vi "Fit Color - Parabolic.vi"(9 "Height":i16, 10 "Color Shadow":u8, 11 "Color Hilite":u8) -> (3 "Polynomial Coefficients":dbl[](array[numeric]))   [LabVIEW 2017, in "Gradient Rectangle.lvclass"]
uses:
  Gradient Rectangle.lvclass
  <vilib>/Analysis/NI_AALPro.lvlib
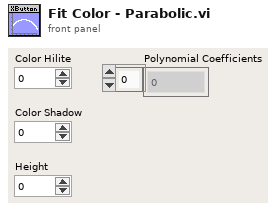
[diagram p1: front panel]
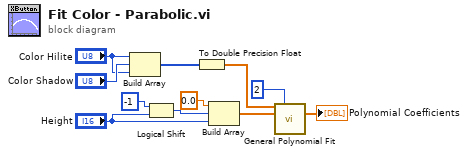
[diagram p0: block diagram]
diagram:
  n1 = Build Array("Color Hilite", "Color Shadow", "Color Hilite") -> (w2:u8[])
  n2 = Logical Shift(y=i16 -1, x="Height") -> (x << y=w5:i16)
  n3 = To Double Precision Float(number=w2) -> (double precision float=w7:dbl[])
  n4 = Build Array(0.0 ("element"), w5, "Height") -> (w6:dbl[])
  n5 = call <vilib>:"General Polynomial Fit.vi"("Y"=w7, "polynomial order"=2, "X"=w6) -> ("Polynomial Coefficients"=→"Polynomial Coefficients":dbl[])  [unwired: 9 in, 3 out]
